vi "Start SLSC FPGA.vi"(8 "error in (no error)":errorcluster, 11 "FPGA Ref in":refnum<k20>) -> (0 "error out":errorcluster, 3 "FPGA Ref out":refnum<k20>)   [LabVIEW 2014, in "SLSC configuration Engine.lvlib"]
uses:
  SLSC configuration Engine.lvlib
  <vilib>/NI/LVFPGA Adv Session Resources/OpenByNameSubVI.vi
  Shared/Constants.vi
  <vilib>/rvi/interface/common/dynamic/niFpgaEscapeDelimiterAndNull.vi
  <vilib>/Utility/error.llb/Error Cluster From Error Code.vi
  <vilib>/rvi/errors/niLvFpgaAdjustHostInterfaceError.vi
  <vilib>/NI/LVFPGA Adv Session Resources/OpenByName.xnode
  <vilib>/rvi/interface/nirviReadWriteControl/nirviReadWriteControl.xnode
  Shared/SLSC configuration Shared.lvlib
  NiFpgaLv.dll
  <vilib>/rvi/interface/Simulation/niFpgaSimulationCallBeginRW.vi
  <vilib>/NI/LVFPGA Adv Session Resources/LVFPGAAdvSessionResources.lvlib
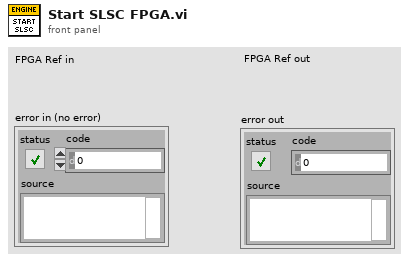
[diagram p1: front panel]
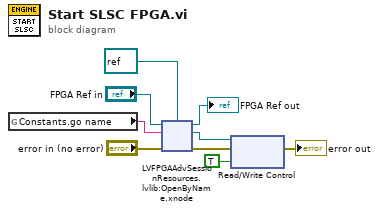
[diagram p0: block diagram]
diagram:
  n1 = global read "Constants.vi" "Constants.go name"() -> (w5:string)
  n2 = xnode "LVFPGAAdvSessionResources.lvlib:OpenByName.xnode"("FPGA VI Reference in"="FPGA Ref in", "Resource name in"=w5, "Single resource reference type in"=refnum<k20> refnum ("Single resource reference out"), "Error in"="error in (no error)") -> ("Single resource reference out"=w7:refnum<k20>, "Error out"=w9:errorcluster, "FPGA VI Reference out"=→"FPGA Ref out":refnum<k20>)
  n3 = xnode "Read/Write Control"("FPGA VI Reference In"=w7, "error in"=w9, "Value"=TRUE) -> ("error out"=→"error out":errorcluster)  [unwired: 1 out]
